vi "Write to File.vi"(8 "error in (no error)":errorcluster, 11 "Report":refnum<class "Report.lvclass">) -> (0 "error out":errorcluster, 3 "Report out":refnum<class "Report.lvclass">)   [LabVIEW 2009, in "Report.lvclass"]
doc: "This VI is overriden by child methods which write the object data to file\\ for the corresponding child class.\n\nAAL 9/09"
uses:
  Report.lvclass
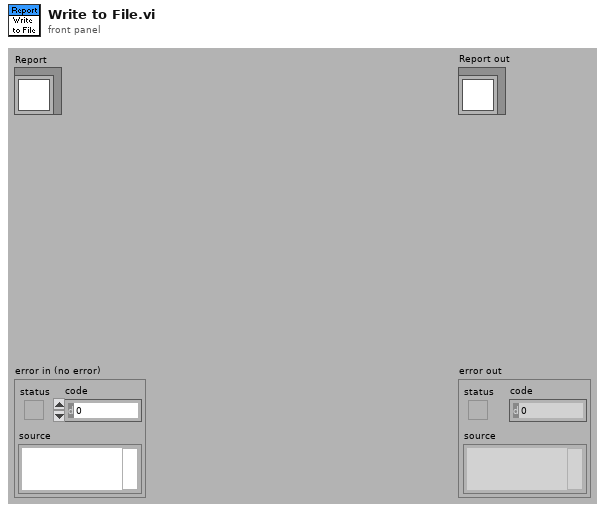
[diagram p1: front panel]
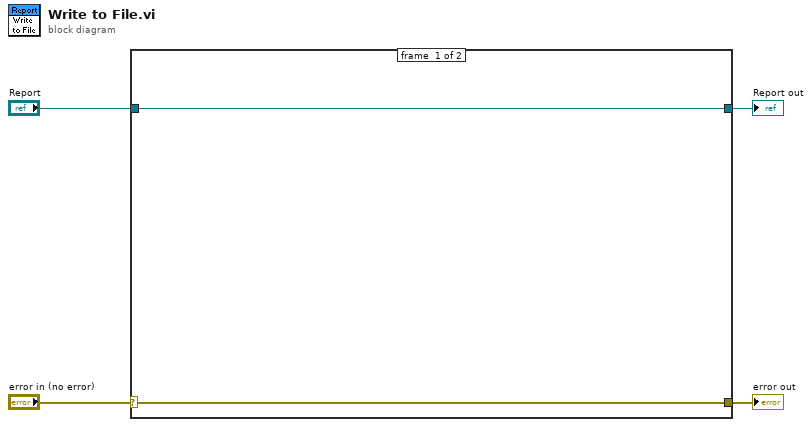
[diagram p0: block diagram]
diagram:
  n1 = case shown="No Error" "error in (no error)" {
    selector: "error in (no error)" -> [w5 w8]
    tunnel: [w5 w8] -> w3
    tunnel: [w6 w7] -> w2
    tunnel: "Report" -> [w6 w7]
    frame #0 {
    }
    frame #1 {
    }
  }
  "error out" <- w3
  "Report out" <- w2
